vi "ConigureHW.vi"(8 "error in (no error)":errorcluster, 11 "BME_DG_System in":refnum<class "BME_DG_System.lvclass">) -> (0 "error out":errorcluster, 3 "BME_DG_System out":refnum<class "BME_DG_System.lvclass">)   [LabVIEW 2009, in "POLARIS BME DG.lvlib" / "BME_DG_System.lvclass"]
doc: "VI calls BME_DG_Base:ConfigHW.vi for each DG object. Over dynamic dispatch mechanism the proper ConfigHW.vi of inheriting class will be called.\n \nCall this VI after error free system initialization from configuration file.\n\n---------------\n\nauthor: Alexander Kessler, Helmholtz-Institut-Jena \nmaintainer: Alexander Kessler: alexander.kessler@uni-jena.de\n\n\nLicense Agreement for this software:\n\nCopyright (C)\nHelmholtz-Institut-Jena\nFröbelsteg 3\n07743 Jena\nGermany\n\nContact: alexander.kessler@uni-jena.de\n\nThis program is free software; you can redistribute it and/or modify it under the terms of the GNU General Public License as published by the Free Software Foundation; either version 2 of the license, or (at your option) any later version.\n\nThis program is distributed in the hope that it will be useful, but WITHOUT ANY WARRANTY; without even the implied warranty of MERCHANTABILITY or FITNESS FOR A PARTICULAR PURPOSE. See the GNU General License for more details (http://www.gnu.org)."
uses:
  BME_DG_System.lvclass
  BME_DG_System.lvclass/BME_DG_System.ctl
  BME_DG_Base/BME_DG_Base.lvclass
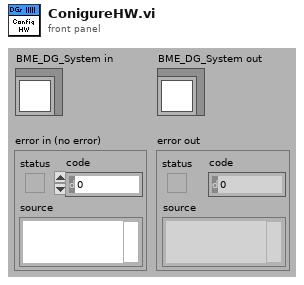
[diagram p1: front panel]
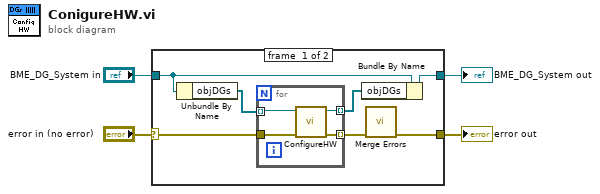
[diagram p0: block diagram]
diagram:
  n1 = case shown="No Error" "error in (no error)" {
    selector: "error in (no error)" -> [w9 w17]
    tunnel: [w5 w17] -> w3
    tunnel: [w8 w16] -> w1
    tunnel: "BME_DG_System in" -> [w11 w16]
    frame #0 {
      n2 = Unbundle By Name(w11) -> ("objDGs"=w10:refnum<class "BME_DG_Base.lvclass">[])
      n3 = for {
        tunnel: w10 -> [w15] mode=indexing
        tunnel: w9 -> [w14]
        tunnel: [w13] -> w6 mode=indexing
        tunnel: [w12] -> w7 mode=indexing
        n4 = call "ConfigureHW.vi"("error in (no error)"=w14, "BME_DG_Base in"=w15) -> ("error out"=w13:errorcluster, "BME_DG_Base out"=w12:refnum<class "BME_DG_Base.lvclass">)  [unwired: 8 in]
      }
      n5 = Bundle By Name(cluster=w11, "objDGs"=w7) -> (w8:refnum<class "BME_DG_System.lvclass">)
      n6 = call <vilib>:"Merge Errors.vi"("error array in"=w6) -> ("error out"=w5:errorcluster)  [unwired: 6 in]
    }
    frame #1 {
    }
  }
  "error out" <- w3
  "BME_DG_System out" <- w1
